vi "New Log File.vi"(3 "error in (no error)":errorcluster) -> (8 "refnum out":refnum<file>)   [LabVIEW 2014]
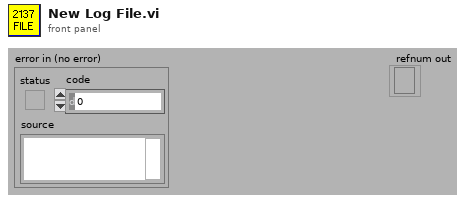
[diagram p1: front panel]
types:
  T1 = enum16{"open", "replace", "create", "open or create", "replace or create", "replace or create with confirmation"}
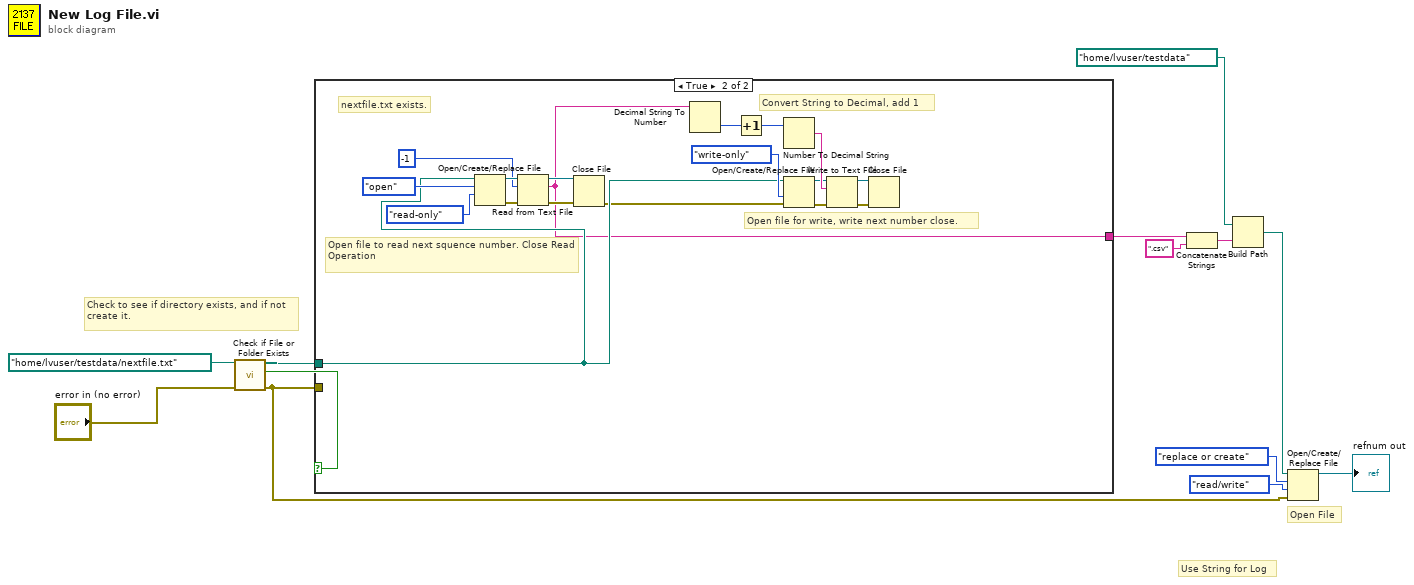
[diagram p0: block diagram]
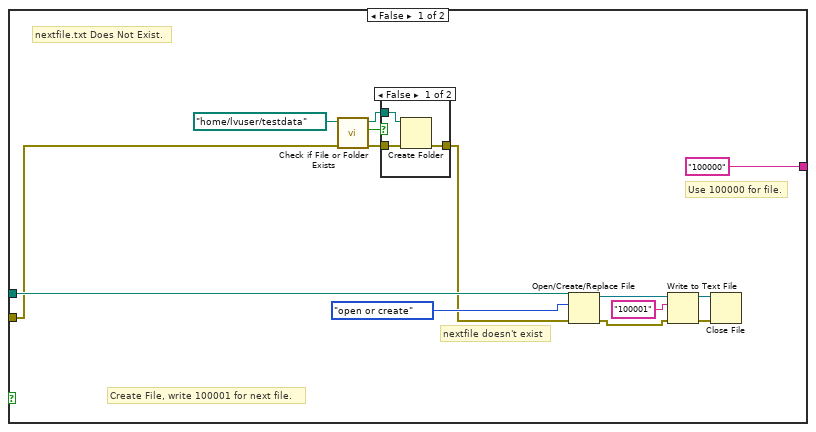
[diagram p2: hidden frame]
diagram:
  # "Use String for Log"
  # "Open File"
  # "Check to see if directory exists, and if not create it."
  n1 = call <vilib>:"Check if File or Folder Exists.vi"("error in (no error)"="error in (no error)", "path"=path "/home/lvuser/testdata/nextfile.txt" ("path (use dialog)")) -> ("error out"=w1:errorcluster, "file or folder exists?"=w9:bool, "dup path"=w8:path)  [unwired: 7 in]
  n2 = case shown="True" w9 {
    tunnel: w8 -> [w26 w36]
    tunnel: ["100000" w32] -> w5
    tunnel: w1 -> [w14 _]
    frame False {
      # "nextfile.txt Does Not Exist."
      # "Use 100000 for file."
      # "Create File, write 100001 for next file."
      # "nextfile doesn't exist"
      n3 = call <vilib>:"Check if File or Folder Exists.vi"("error in (no error)"=w14, "path"=path "/home/lvuser/testdata") -> ("error out"=w20:errorcluster, "file or folder exists?"=w15:bool, "dup path"=w19:path)  [unwired: 7 in]
      n4 = case shown="False" w15 {
        tunnel: w20 -> [w29 w31]
        tunnel: w19 -> [w28 _]
        tunnel: [w30 w31] -> w17
        frame False {
          n5 = Create Folder(path (use dialog)=w28, error in=w29) -> (error out=w30:errorcluster)  [unwired: 1 in, 2 out]
        }
        frame True {
        }
      }
      n6 = Open/Create/Replace File(file path (use dialog)=w26, error in=w17, operation (0:open)=T1."open or create") -> (refnum out=w22:refnum<file>, error out=w16:errorcluster)  [unwired: 3 in, 1 out]
      n7 = Write to Text File(file (use dialog)=w22, text="100001", error in=w16) -> (refnum out=w23:refnum<file>, error out=w24:errorcluster)  [unwired: 1 in, 1 out]
      n8 = Close File(refnum=w23, error in=w24) -> ()  [unwired: 2 out]
    }
    frame True {
      # "Open file for write, write next number close."
      # "Convert String to Decimal, add 1"
      # "nextfile.txt exists."
      # "Open file to read next squence number. Close Read Operation"
      n9 = Open/Create/Replace File(file path (use dialog)=w36, operation (0:open)=T1."open", access (0:read/write)=enum16{"read/write", "read-only", "write-only"}."read-only") -> (refnum out=w47:refnum<file>, error out=w46:errorcluster)  [unwired: 1 in, 3 out]
      n10 = Read from Text File(file (use dialog)=w47, count=-1, error in=w46) -> (refnum out=w45:refnum<file>, text=w32:string, error out=w37:errorcluster)  [unwired: 1 in, 1 out]
      n11 = Close File(refnum=w45, error in=w37) -> (error out=w35:errorcluster)  [unwired: 1 out]
      n12 = Decimal String To Number(string=w32) -> (number=w38:i32)  [unwired: 2 in, 1 out]
      n13 = Increment(x=w38) -> (x+1=w43:i32)
      n14 = Number To Decimal String(number=w43) -> (decimal integer string=w42:string)  [unwired: 1 in]
      n15 = Open/Create/Replace File(file path (use dialog)=w36, error in=w35, access (0:read/write)=enum16{"read/write", "read-only", "write-only"}."write-only") -> (refnum out=w41:refnum<file>, error out=w34:errorcluster)  [unwired: 3 in, 1 out]
      n16 = Write to Text File(file (use dialog)=w41, text=w42, error in=w34) -> (refnum out=w39:refnum<file>, error out=w40:errorcluster)  [unwired: 1 in, 1 out]
      n17 = Close File(refnum=w39, error in=w40) -> ()  [unwired: 2 out]
    }
  }
  n18 = Concatenate Strings(w5, ".csv" ("string")) -> (w3:string)
  n19 = Build Path(base path=path "/home/lvuser/testdata", name or relative path=w3) -> (appended path=w12:path)
  n20 = Open/Create/Replace File(file path (use dialog)=w12, error in=w1, operation (0:open)=T1."replace or create", access (0:read/write)=enum16{"read/write", "read-only", "write-only"}."read/write") -> (refnum out=→"refnum out":refnum<file>)  [unwired: 4 out]
